vi "DMM Scan Reset_2_test.vi"(8 "error in (no error)":errorcluster, 10 "VISA in resource name 2":refnum<visa-resource-name>, 11 "VISA in resource name":refnum<visa-resource-name>) -> (0 "error out":errorcluster, 3 "VISA resource name out":refnum<visa-resource-name>)   [LabVIEW 2023]
uses:
  <instrlib>/Agilent 3446X Series/Agilent 3446X Series.lvlib
panel:
  out "error out 2":errorcluster
  out "read buffer":string
  out "error out 4":errorcluster caption="error out"
  out "error out 3":errorcluster
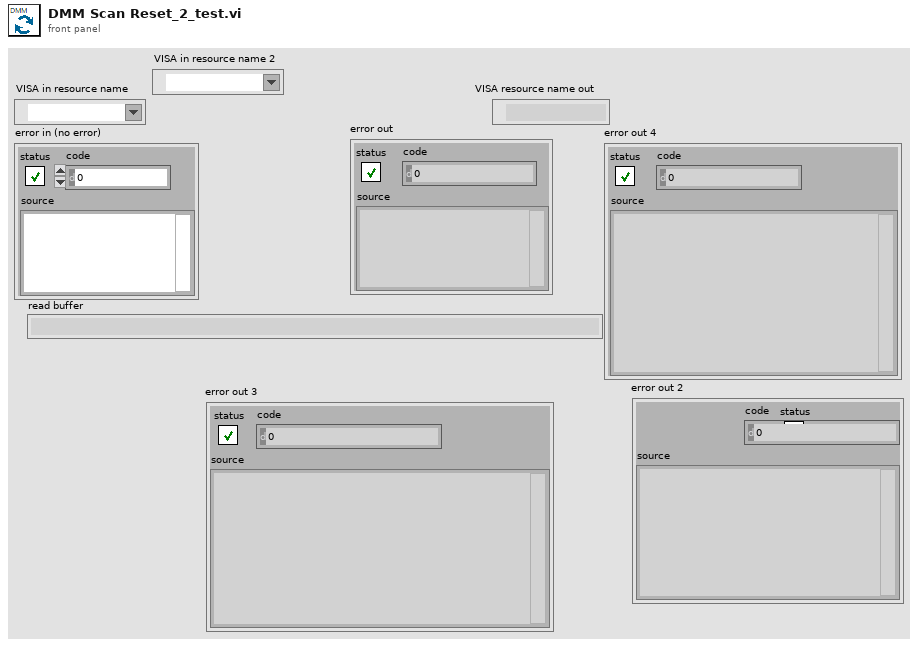
[diagram p1: front panel]
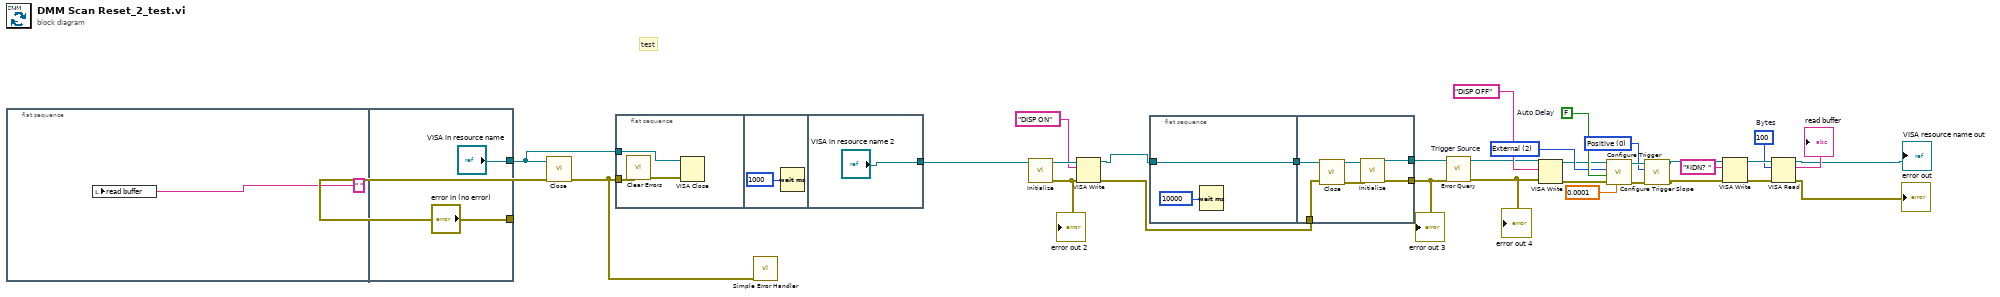
[diagram p0: block diagram]
diagram:
  w17 = u32 100  # Bytes
  w30 = 0 items=["Positive", "Negative"] ("Trigger Edge (1: Negative)")
  w28 = 2 items=["Immediate", "Software (Bus)", "External"]  # Trigger Source
  w29 = FALSE  # Auto Delay
  # "test"
  n1 = flat-sequence {
    tunnel: ["error in (no error)"] -> w23
    tunnel: ["VISA in resource name"] -> w1
    frame #0 {
      n2 = local write "read buffer"(" " ("read buffer")) -> ()
    }
    frame #1 {
    }
  }
  n3 = call <instrlib>:"Close.vi"("error in (no error)"=w23, "VISA resource name"=w1) -> ("error out"=w22:errorcluster)  [unwired: 9 in]
  n4 = flat-sequence {
    tunnel: w22 -> [w38]
    tunnel: w1 -> [w37]
    tunnel: ["VISA in resource name 2"] -> w2
    frame #0 {
      n5 = call <vilib>:"Clear Errors.vi"("error in (no error)"=w38) -> ("error out"=w36:errorcluster)  [unwired: 5 in, 1 out]
      n6 = VISA Close(VISA resource name=w37, error in (no error)=w36) -> ()  [unwired: 1 out]
    }
    frame #1 {
      n7 = Wait (ms)(milliseconds to wait=u32 1000) -> ()  [unwired: 1 out]
    }
    frame #2 {
    }
  }
  n8 = call <vilib>:"Simple Error Handler.vi"("error in (no error)"=w22) -> ()  [unwired: 4 in, 5 out]
  n9 = call <instrlib>:"Initialize.vi"("VISA resource name"=w2) -> ("error out"=w9:errorcluster, "VISA resource name out"=w10:refnum<visa-resource-name>)  [unwired: 4 in, 5 out]
  "error out 2" <- w9
  n10 = VISA Write(VISA resource name=w10, write buffer="DISP ON", error in (no error)=w9) -> (VISA resource name out=w6:refnum<visa-resource-name>, error out=w4:errorcluster)  [unwired: 1 out]
  n11 = flat-sequence {
    tunnel: w6 -> [w42]
    tunnel: [w42] -> w5
    tunnel: [w47] -> w7
    tunnel: w5 -> [w45]
    tunnel: w4 -> [w46]
    tunnel: [w43] -> w3
    frame #0 {
      n12 = Wait (ms)(milliseconds to wait=u32 10000) -> ()  [unwired: 1 out]
    }
    frame #1 {
      n13 = call <instrlib>:"Close.vi"("error in (no error)"=w46, "VISA resource name"=w45) -> ("error out"=w44:errorcluster)  [unwired: 9 in]
      n14 = call <instrlib>:"Initialize.vi"("error in (no error)"=w44, "VISA resource name"=w45) -> ("error out"=w47:errorcluster, "VISA resource name out"=w43:refnum<visa-resource-name>)  [unwired: 3 in, 5 out]
    }
  }
  n15 = call <instrlib>:"Error Query.vi"("error in (no error)"=w7, "VISA resource name"=w3) -> ("error out"=w20:errorcluster, "VISA resource name out"=w21:refnum<visa-resource-name>)  [unwired: 8 out]
  "error out 4" <- w20
  n16 = VISA Write(VISA resource name=w21, write buffer="DISP OFF", error in (no error)=w20) -> (VISA resource name out=w25:refnum<visa-resource-name>, error out=w24:errorcluster)  [unwired: 1 out]
  n17 = call <instrlib>:"Configure Trigger.vi"("Manual Trigger Delay (1 s)"=0.0001, "error in (no error)"=w24, "Auto Delay (F:Disable)"=w29, "Trigger Source (0: Immediate)"=w28, "VISA resource name"=w25) -> ("error out"=w32:errorcluster, "VISA resource name out"=w31:refnum<visa-resource-name>)  [unwired: 1 in, 4 out]
  n18 = call <instrlib>:"Configure Trigger Slope.vi"("error in (no error)"=w32, "Trigger Edge (1: Negative)"=w30, "VISA resource name"=w31) -> ("error out"=w13:errorcluster, "VISA resource name out"=w14:refnum<visa-resource-name>)  [unwired: 7 in]
  n19 = VISA Write(VISA resource name=w14, write buffer="*IDN? ", error in (no error)=w13) -> (VISA resource name out=w18:refnum<visa-resource-name>, error out=w19:errorcluster)  [unwired: 1 out]
  n20 = VISA Read(VISA resource name=w18, byte count=w17, error in (no error)=w19) -> (VISA resource name out=→"VISA resource name out":refnum<visa-resource-name>, read buffer=→"read buffer":string, error out=→"error out":errorcluster)  [unwired: 1 out]
  "error out 3" <- w7
